vi "Gunsim.vi"(8 "error in (no error)":errorcluster, 9 "Parameters":T1={"Framerate"=1000, "Initial Velocity(ft/s)"=40.0, "Max Angle"=60, "Min Angle"=0, "Sims/angle"=10, "Full Path"=path "", "Partial Path"=path ""}, 10 "Other Constants":T3={"Ball Diameter(in)"=10.0, "Air Density(g/in^3)"=0.02, "Drag coefficient"=0.5, "Ball Mass(g)"=300.0, "gravity(in/s^2)"=-386.09, "Minimum Goal Height(in)"=90.0, "Maximum Goal Height(in)"=104.0}, 11 "Robot Constants":T2={"Distance from Pivot Point to Drive Mount(in)"=16.25, "Distance from Pivot Point to Arm Mount(in)"=5.625, "Distance from Pivot Point to Launcher(in)"=31.125, "Distance from Pivot Point to Camera(in)"=25.625, "WheelEncoder Ticks/Revolution"=2048.0, "Wheel Radius"=4.0, "Triangle Angle(degrees)"=51.75, "Minimum LA Distance(inches)"=12.125, "LA Distance/Tick(inches)"=-64.0}) -> (0 "error out":errorcluster, 2 "Full Sheet":dbl[][](array[numeric]), 3 "Trimmed Sheet":dbl[][](array[numeric]))   [LabVIEW 2015]
uses:
  Robot Global Data.vi
  <vilib>/Utility/file.llb/Write Delimited Spreadsheet (DBL).vi
panel:
  out "RPM":dbl
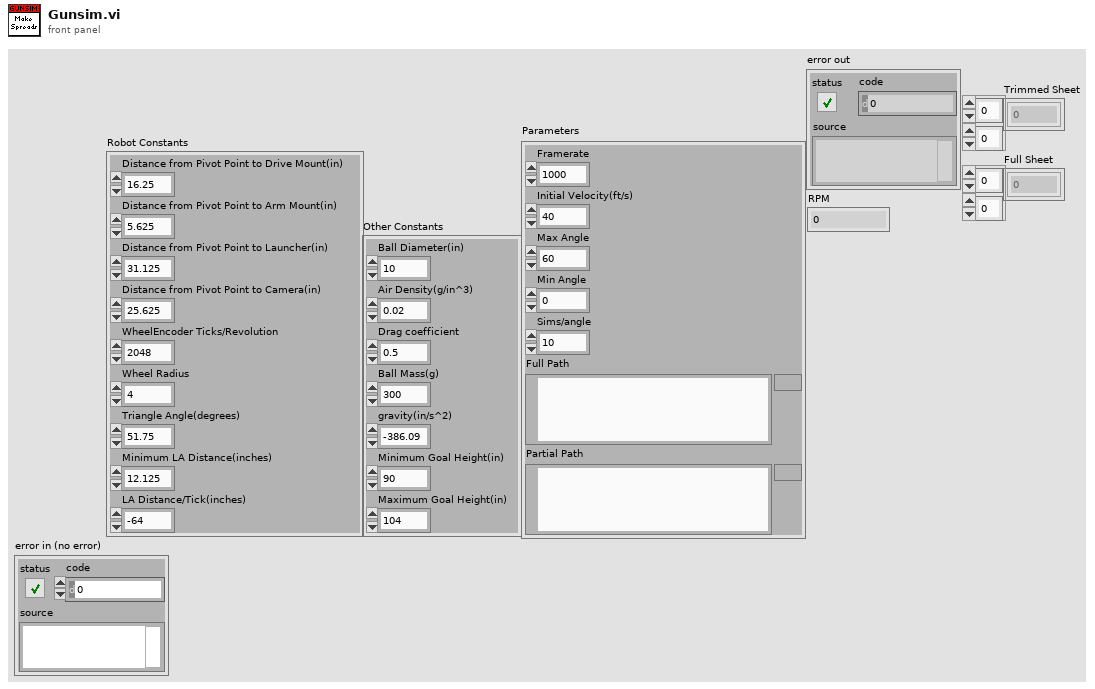
[diagram p1: front panel]
types:
  T1 = cluster{"Framerate":i32, "Initial Velocity(ft/s)":dbl, "Max Angle":i32, "Min Angle":i32, "Sims/angle":i32, "Full Path":path, "Partial Path":path}
  T2 = cluster{"Distance from Pivot Point to Drive Mount(in)":dbl, "Distance from Pivot Point to Arm Mount(in)":dbl, "Distance from Pivot Point to Launcher(in)":dbl, "Distance from Pivot Point to Camera(in)":dbl, "WheelEncoder Ticks/Revolution":dbl, "Wheel Radius":dbl, "Triangle Angle(degrees)":dbl, "Minimum LA Distance(inches)":dbl, "LA Distance/Tick(inches)":dbl}
  T3 = cluster{"Ball Diameter(in)":dbl, "Air Density(g/in^3)":dbl, "Drag coefficient":dbl, "Ball Mass(g)":dbl, "gravity(in/s^2)":dbl, "Minimum Goal Height(in)":dbl, "Maximum Goal Height(in)":dbl}
  T4 = cluster{"Drag":dbl, "gravity(in/s^2)":dbl, "Minimum Goal Height(in)":dbl, "Maximum Goal Height(in)":dbl, "xspeed":dbl, "yspeed":dbl, "xpos":dbl, "ypos":dbl, "Frametime":dbl, "Output Array":dbl[]}
  T5 = cluster{"Firing Angle":dbl, "Initial Velocity":dbl}
  T6 = cluster{"Minimum Distance":dbl, "Ideal Distance":dbl, "Viable Distances":dbl[], "Maximum Distance":dbl}
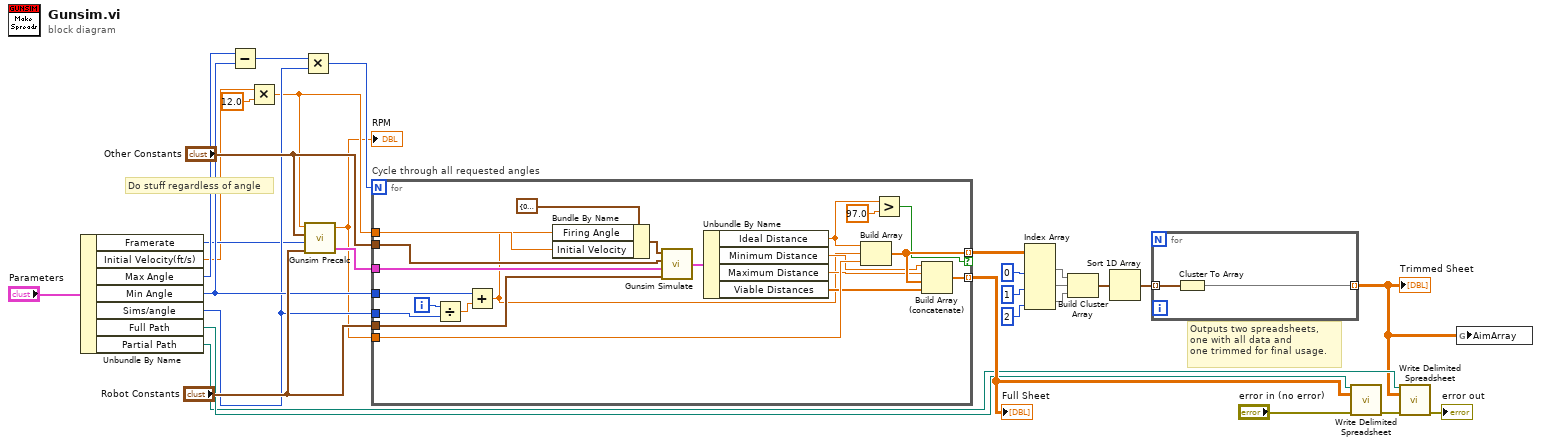
[diagram p0: block diagram]
diagram:
  # "Do stuff regardless of angle"
  # "Outputs two spreadsheets,\none with all data and \none trimmed for final usage."
  n1 = Unbundle By Name("Parameters") -> ("Framerate"=w10:i32, "Initial Velocity(ft/s)"=w4:dbl, "Max Angle"=w13:i32, "Min Angle"=w12:i32, "Sims/angle"=w11:i32, "Full Path"=w9:path, "Partial Path"=w8:path)
  n2 = Subtract(x=w13, y=w12) -> (x-y=w30:i32)
  n3 = Multiply(x=w4, y=12.0) -> (x*y=w3:dbl)
  n4 = Multiply(x=w30, y=w11) -> (x*y=w29:i32)
  n5 = call "Gunsim Precalc.vi"("Robot Constants"="Robot Constants", "Framerate"=w10, "Other Constants"="Other Constants", "Initial Velocity(in/s)"=w3) -> ("output cluster"=w28:T4, "RPM"=w2:dbl)  [unwired: 1 in]
  "RPM" <- w2
  n6 = for "Cycle through all requested angles" {
    N: w29 -> [_]
    tunnel: w12 -> [w51]
    tunnel: w3 -> [w47]
    tunnel: [w38] -> w24 mode=indexing if=w31
    tunnel: w11 -> [w46]
    tunnel: w2 -> [w43]
    tunnel: w28 -> [w42]
    tunnel: "Robot Constants" -> [w41]
    tunnel: "Other Constants" -> [w40]
    tunnel: [w37] -> w25 mode=indexing
    i -> [w45]
    n7 = Divide(x=w45, y=w46) -> (x/y=w44:dbl)
    n8 = Add(x=w51, y=w44) -> (x+y=w34:dbl)
    n9 = Bundle By Name(cluster=T5 {"Firing Angle"=0.0, "Initial Velocity"=0.0} ("Parameters"), "Firing Angle"=w34, "Initial Velocity"=w47) -> (w50:T5)
    n10 = call "Gunsim Simulate.vi"("Robot Constants"=w41, "cluster in"=w42, "Other Constants"=w40, "Parameters"=w50) -> ("Range"=w48:T6)
    n11 = Unbundle By Name(w48) -> ("Ideal Distance"=w32:dbl, "Minimum Distance"=w35:dbl, "Maximum Distance"=w36:dbl, "Viable Distances"=w39:dbl[])
    n12 = Build Array(w32, w34, w43) -> (w38:dbl[])
    n13 = Greater?(x=w32, y=97.0) -> (0:w31:bool)
    n14 = Build Array (concatenate)(w35, w36, w38, w39) -> (w37:dbl[])
  }
  "Full Sheet" <- w25
  n15 = Index Array(array=w24, index (col) #1=0 ("index"), index (col) #2=1 ("index"), index (col) #3=2 ("index")) -> (element #1=w20:dbl[], element #2=w19:dbl[], element #3=w18:dbl[])  [unwired: 3 in]
  n16 = Build Cluster Array(w20, w19, w18) -> (w17:cluster{"RPM":dbl, "RPM":dbl, "RPM":dbl}[])
  n17 = Sort 1D Array(array=w17) -> (sorted array=w16:cluster{"RPM":dbl, "RPM":dbl, "RPM":dbl}[])
  n18 = for {
    tunnel: w16 -> [w53] mode=indexing
    tunnel: [w52] -> w1 mode=indexing
    n19 = Cluster To Array(cluster=w53) -> (array=w52:dbl[])
  }
  "Trimmed Sheet" <- w1
  n20 = call-poly <vilib>:"Write Delimited Spreadsheet.vi"("file path (dialog if empty)"=w9, "2D data"=w25, "error in (no error)"="error in (no error)") -> ("error out"=w15:errorcluster)  [unwired: 11 in, 1 out]
  n21 = call-poly <vilib>:"Write Delimited Spreadsheet.vi"("file path (dialog if empty)"=w8, "2D data"=w1, "error in (no error)"=w15) -> ("error out"=→"error out":errorcluster)  [unwired: 11 in, 1 out]
  n22 = global write "Robot Global Data.vi" "AimArray"(w1) -> ()
